vi "data types.vi"() -> ()   [LabVIEW 2019]
panel:
  out "Error Out":errorcluster
  in  "TDMS File":path=path "C:/Python/projects/nitdms/tests/tdms_files/data types.tdms"
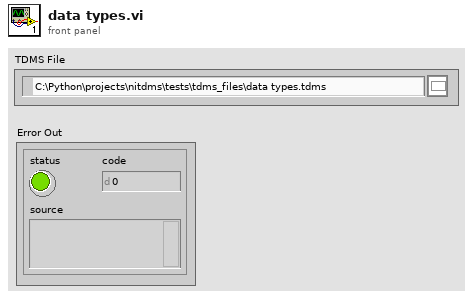
[diagram p1: front panel]
types:
  T1 = enum16{"open", "open or create", "create or replace", "create", "open (read-only)"}
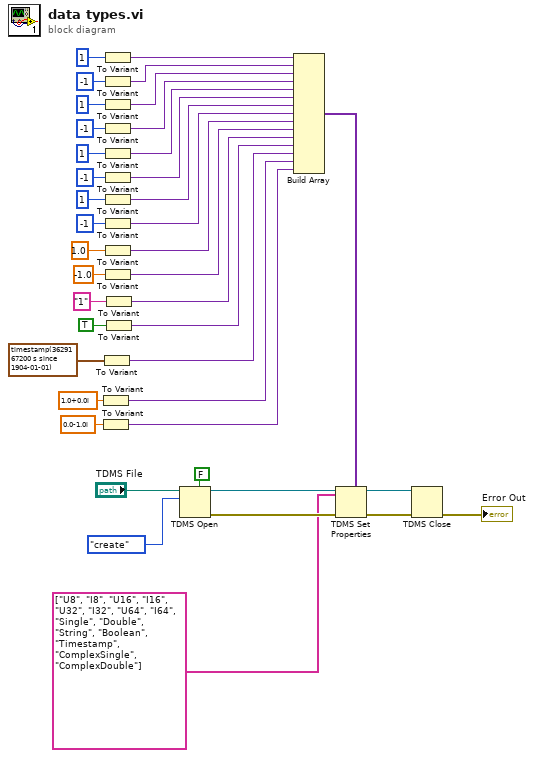
[diagram p0: block diagram]
diagram:
  n1 = To Variant(anything=csg 1.0+0.0i) -> (Variant=w2:variant)
  n2 = To Variant(anything=cdb 0.0-1.0i) -> (Variant=w1:variant)
  n3 = To Variant(anything=timestamp(3629167200 s since 1904-01-01)) -> (Variant=w5:variant)
  n4 = To Variant(anything=u8 1) -> (Variant=w31:variant)
  n5 = To Variant(anything=i8 -1) -> (Variant=w30:variant)
  n6 = To Variant(anything=u16 1) -> (Variant=w20:variant)
  n7 = To Variant(anything=i16 -1) -> (Variant=w19:variant)
  n8 = To Variant(anything=u32 1) -> (Variant=w18:variant)
  n9 = To Variant(anything=-1) -> (Variant=w17:variant)
  n10 = To Variant(anything=u64 1) -> (Variant=w16:variant)
  n11 = To Variant(anything=i64 -1) -> (Variant=w15:variant)
  n12 = To Variant(anything=sgl 1.0) -> (Variant=w12:variant)
  n13 = To Variant(anything=-1.0) -> (Variant=w11:variant)
  n14 = To Variant(anything="1") -> (Variant=w8:variant)
  n15 = To Variant(anything=TRUE) -> (Variant=w7:variant)
  n16 = TDMS Open(5:FALSE ("create index file? (T)"), 10:T1."create" ("operation (0:open)"), 11:"TDMS File") -> (0:w36:errorcluster, 3:w35:refnum<k34>)  [unwired: 4 in]
  n17 = Build Array(w31, w30, w20, w19, w18, w17, w16, w15, w12, w11, w8, w7, w5, w2, w1) -> (w29:variant[])
  n18 = TDMS Set Properties(5:w29, 7:string[] ["U8", "I8", "U16", "I16", "U32", "I32", "U64", "I64", "Single", "Double", "String", "Boolean", "Timestamp", "ComplexSingle", "ComplexDouble"] ("property names"), 8:w36, 11:w35) -> (0:w28:errorcluster, 3:w27:refnum<k34>)  [unwired: 2 in, 2 out]
  n19 = TDMS Close(8:w28, 11:w27) -> (0:→"Error Out":errorcluster)  [unwired: 1 out]
